vi "Configure Acquisition.vi"(8 "error in":errorcluster, 11 "Scope PXI CFG in":refnum<class "Scope PXI CFG.lvclass">) -> (0 "error out":errorcluster, 3 "Scope PXI CFG out":refnum<class "Scope PXI CFG.lvclass">)   [LabVIEW 2023, in "Scope.lvlib" / "Scope PXI.lvlib" / "Scope PXI CFG.lvclass"]
uses:
  Scope PXI CFG.lvclass
  <instrlib>/niScope/Controls/niScope acquisition type.ctl
  Scope PXI CFG.lvclass/Scope PXI CFG.ctl
  Configuration Base/Configuration Base.lvclass/Configuration Base.ctl
  33e6a676-ff2b-4197-9c74-0448942d65be.vi
  <vilib>/JDP Science/JSONtext/Next JSON Value.vi
  <vilib>/JDP Science/JSONtext/String Subset.vi
  <vilib>/JDP Science/JSONtext/Parsing/Advance past next JSON Value (inlined COPY).vi
  <vilib>/JDP Science/JSONtext/Parsing/Advance past whitespace.vi
  <vilib>/JDP Science/JSONtext/Parsing/Advance past String.vi
  <vilib>/JDP Science/JSONtext/Parsing/Advance past Number.vi
  <vilib>/JDP Science/JSONtext/Parsing/Advance past Line Ending.vi
  <vilib>/JDP Science/JSONtext/Parsing/Parse Full Path or Item Name.vi
  <vilib>/JDP Science/JSONtext/Parsing/Advance past Array.vi
  <vilib>/JDP Science/JSONtext/Parsing/Advance past Object.vi
  <vilib>/JDP Science/JSONtext/support/Error Cluster From Code.vi
  <vilib>/JDP Science/JSONtext/Offset/Find Item Locations by Path.vi
  <vilib>/JDP Science/JSONtext/JSON text to Variant.vi
  <vilib>/Utility/error.llb/Error Cluster From Error Code.vi
  <vilib>/JDP Science/JSONtext/LVClass Serializer/JSONtext LVClass Serializer.lvclass
  <vilib>/ErrorRing/Error Ring.xnode
  Configuration Base/Configuration Base.lvclass
  <vilib>/JDP Science/JSONtext/JSONtext.lvlib
  D:/git/HAL/Configuration Base/Configuration Base.lvclass
  D:/git/HAL/Interfaces/IConfigure/IConfigure.lvclass
  D:/git/HAL/Scope PXI/Scope PXI CFG/Scope PXI CFG.lvclass
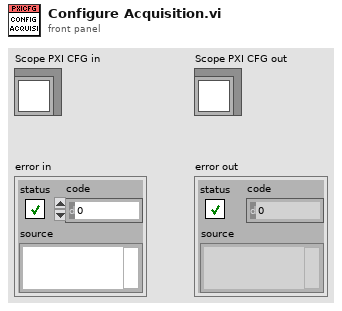
[diagram p1: front panel]
types:
  T1 = typedef "niScope acquisition type.ctl" = i32
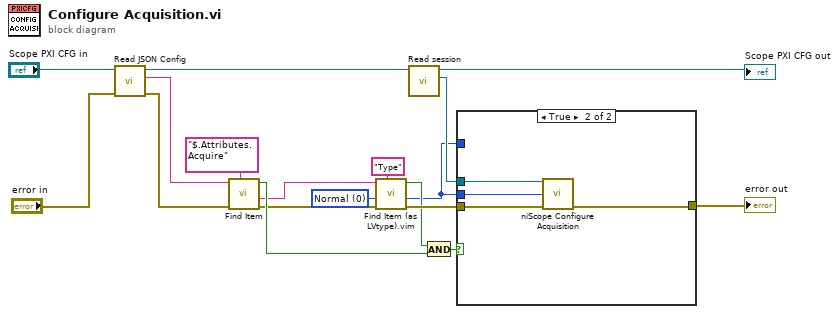
[diagram p0: block diagram]
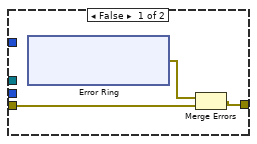
[diagram p2: hidden frame]
diagram:
  w1 = T1 0 items=["Normal"=0, "Flex Res"=1, "DDC"=3] ("acquisition Type")
  n1 = call "Read JSON Config.vi"("error in"="error in", "object in"="Scope PXI CFG in") -> ("error out"=w16:errorcluster, "<JSON>Config"=w17:string, "object out"=w18:refnum<class "Scope PXI CFG.lvclass">)  [unwired: 7 in]
  n2 = call <vilib>:"Find Item.vi"("$Path or Item Name"="$.Attributes.Acquire", "error in (no error)"=w16, "JSON"=w17) -> ("error out"=w13:errorcluster, "<JSON>"=w9:string, "Found"=w15:bool)  [unwired: 5 in, 1 out]
  n3 = call "Find Item (as LVtype).vim"("$Path or Item Name"="Type", "error in (no error)"=w13, "Data Type and Default Value"=w1, "JSON"=w9) -> ("error out"=w10:errorcluster, "Data"=w6:T1, "Found"=w8:bool)  [unwired: 4 in, 1 out]
  n4 = call "Read session.vi"("Scope PXI CFG in"=w18) -> ("session"=w12:refnum<k15>, "Scope PXI CFG out"=→"Scope PXI CFG out":refnum<class "Scope PXI CFG.lvclass">)  [unwired: 8 in, 1 out]
  n5 = And(x=w8, y=w15) -> (x .and. y?=w7:bool)
  n6 = case shown="True" w7 {
    tunnel: w12 -> [_ w28]
    tunnel: w10 -> [w20 w30]
    tunnel: w6 -> [_ w27]
    tunnel: w6 -> [_ _]
    tunnel: [w19 w29] -> w3
    frame False {
      n7 = xnode "Error Ring"() -> ("error out"=w21:errorcluster)
      n8 = Merge Errors(w21, w20) -> (w19:errorcluster)
    }
    frame True {
      n9 = call <instrlib>:"niScope Configure Acquisition.vi"("instrument handle"=w28, "acquisition Type"=w27, "error in"=w30) -> ("error out"=w29:errorcluster)  [unwired: 11 in, 1 out]
    }
  }
  "error out" <- w3
